vi "Parse Ardiuno Q Cmd.vi"(8 "error in":errorcluster, 11 "Q cmd response":string) -> (0 "error out":errorcluster, 2 "pos":i32, 3 "m":i32)   [LabVIEW 2024, in "FW Arduino Control.lvclass"]
uses:
  FW Arduino Control.lvclass
  <vilib>/regexp/Match Regular Expression.xnode
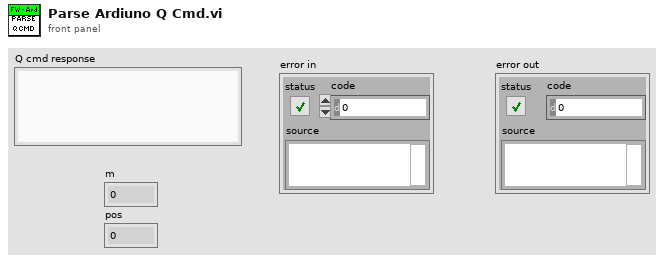
[diagram p1: front panel]
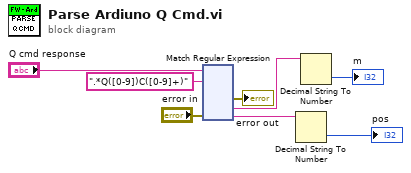
[diagram p0: block diagram]
diagram:
  n1 = xnode "Match Regular Expression"("input string"="Q cmd response", "regular expression"=".*Q([0-9])C([0-9]+)", "error in"="error in") -> ("error out"=→"error out":errorcluster, "submatch 1"=w6:string, "submatch 2"=w4:string)  [unwired: 3 in, 4 out]
  n2 = Decimal String To Number(string=w4) -> (number=→"pos":i32)  [unwired: 2 in, 1 out]
  n3 = Decimal String To Number(string=w6) -> (number=→"m":i32)  [unwired: 2 in, 1 out]
